vi "PyroAnalyze.vi"() -> ()   [LabVIEW 2014]
panel:
  out "Layer":i32
  out "Point":i32
  out "AllStacked":dbl[][][][](array[numeric])
  in  "Save Folder":path
  in  "StackAll":bool
  in  "Add":bool
  in  "Points":cluster{"X":dbl, "Y":dbl}[](array[cluster])
  in  "Size":u8
  in  "Save":bool
  in  "LayAvg":u16
  out "StackedAvg":u16[][][](array[numeric])
  in  "Stack":bool
  in  "Angle":dbl
  out "Image":dbl[][](graph)
  in  "ToImage":bool
  in  "NumPix":dbl
  in  "Width(mm)":dbl
  in  "Point1":cluster{"X":dbl, "Y":dbl}
  in  "Set1":bool
  out "Plot":cluster{"X":i16[], "Y":i16[]}(graph)
  in  "Deci":i32=5
  in  "Index":u32
  in  "Load":bool
  in  "Folder":path
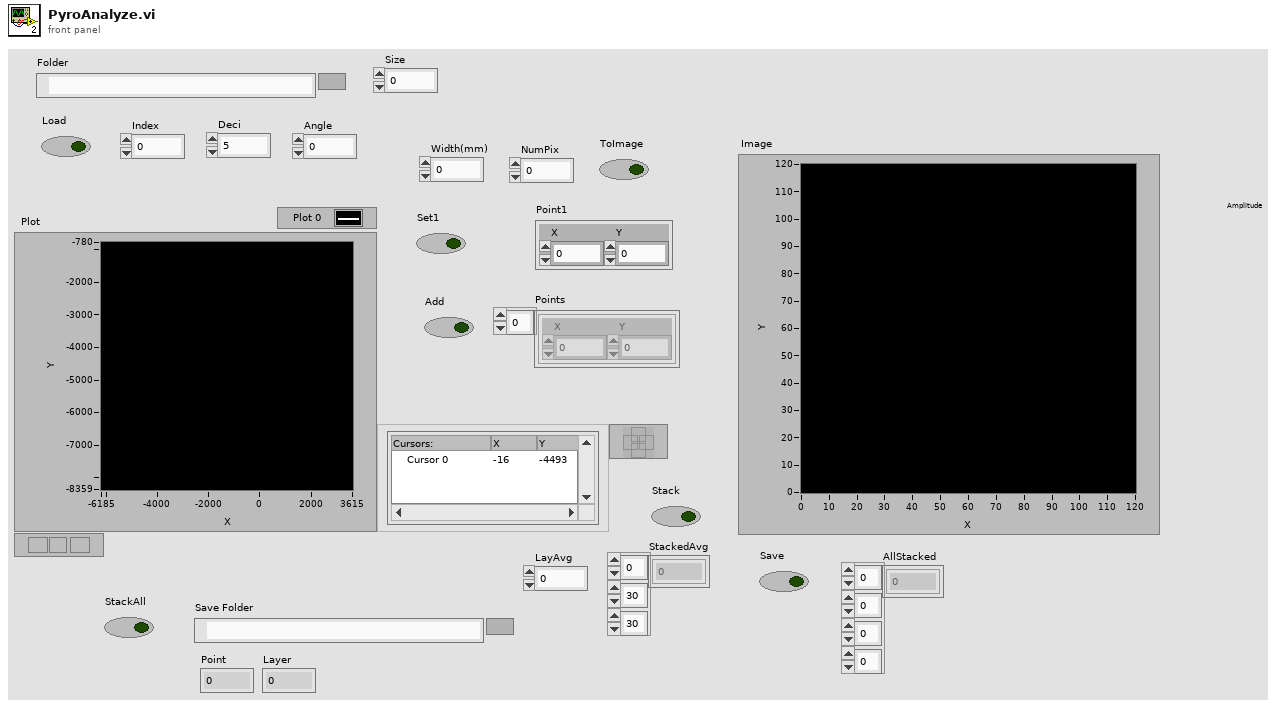
[diagram p1: front panel]
types:
  T1 = typedef "LVPointDoubleTypeDef.ctl" = cluster{"Cursor X":dbl, "Cursor Y":dbl}
  T2 = typedef "imagedata.ctl" = cluster{"image type":i32, "image depth":i32, "image":u8[], "mask":u8[], "colors":u32[], "Rectangle":cluster{"left":i16, "top":i16, "right":i16, "bottom":i16}}
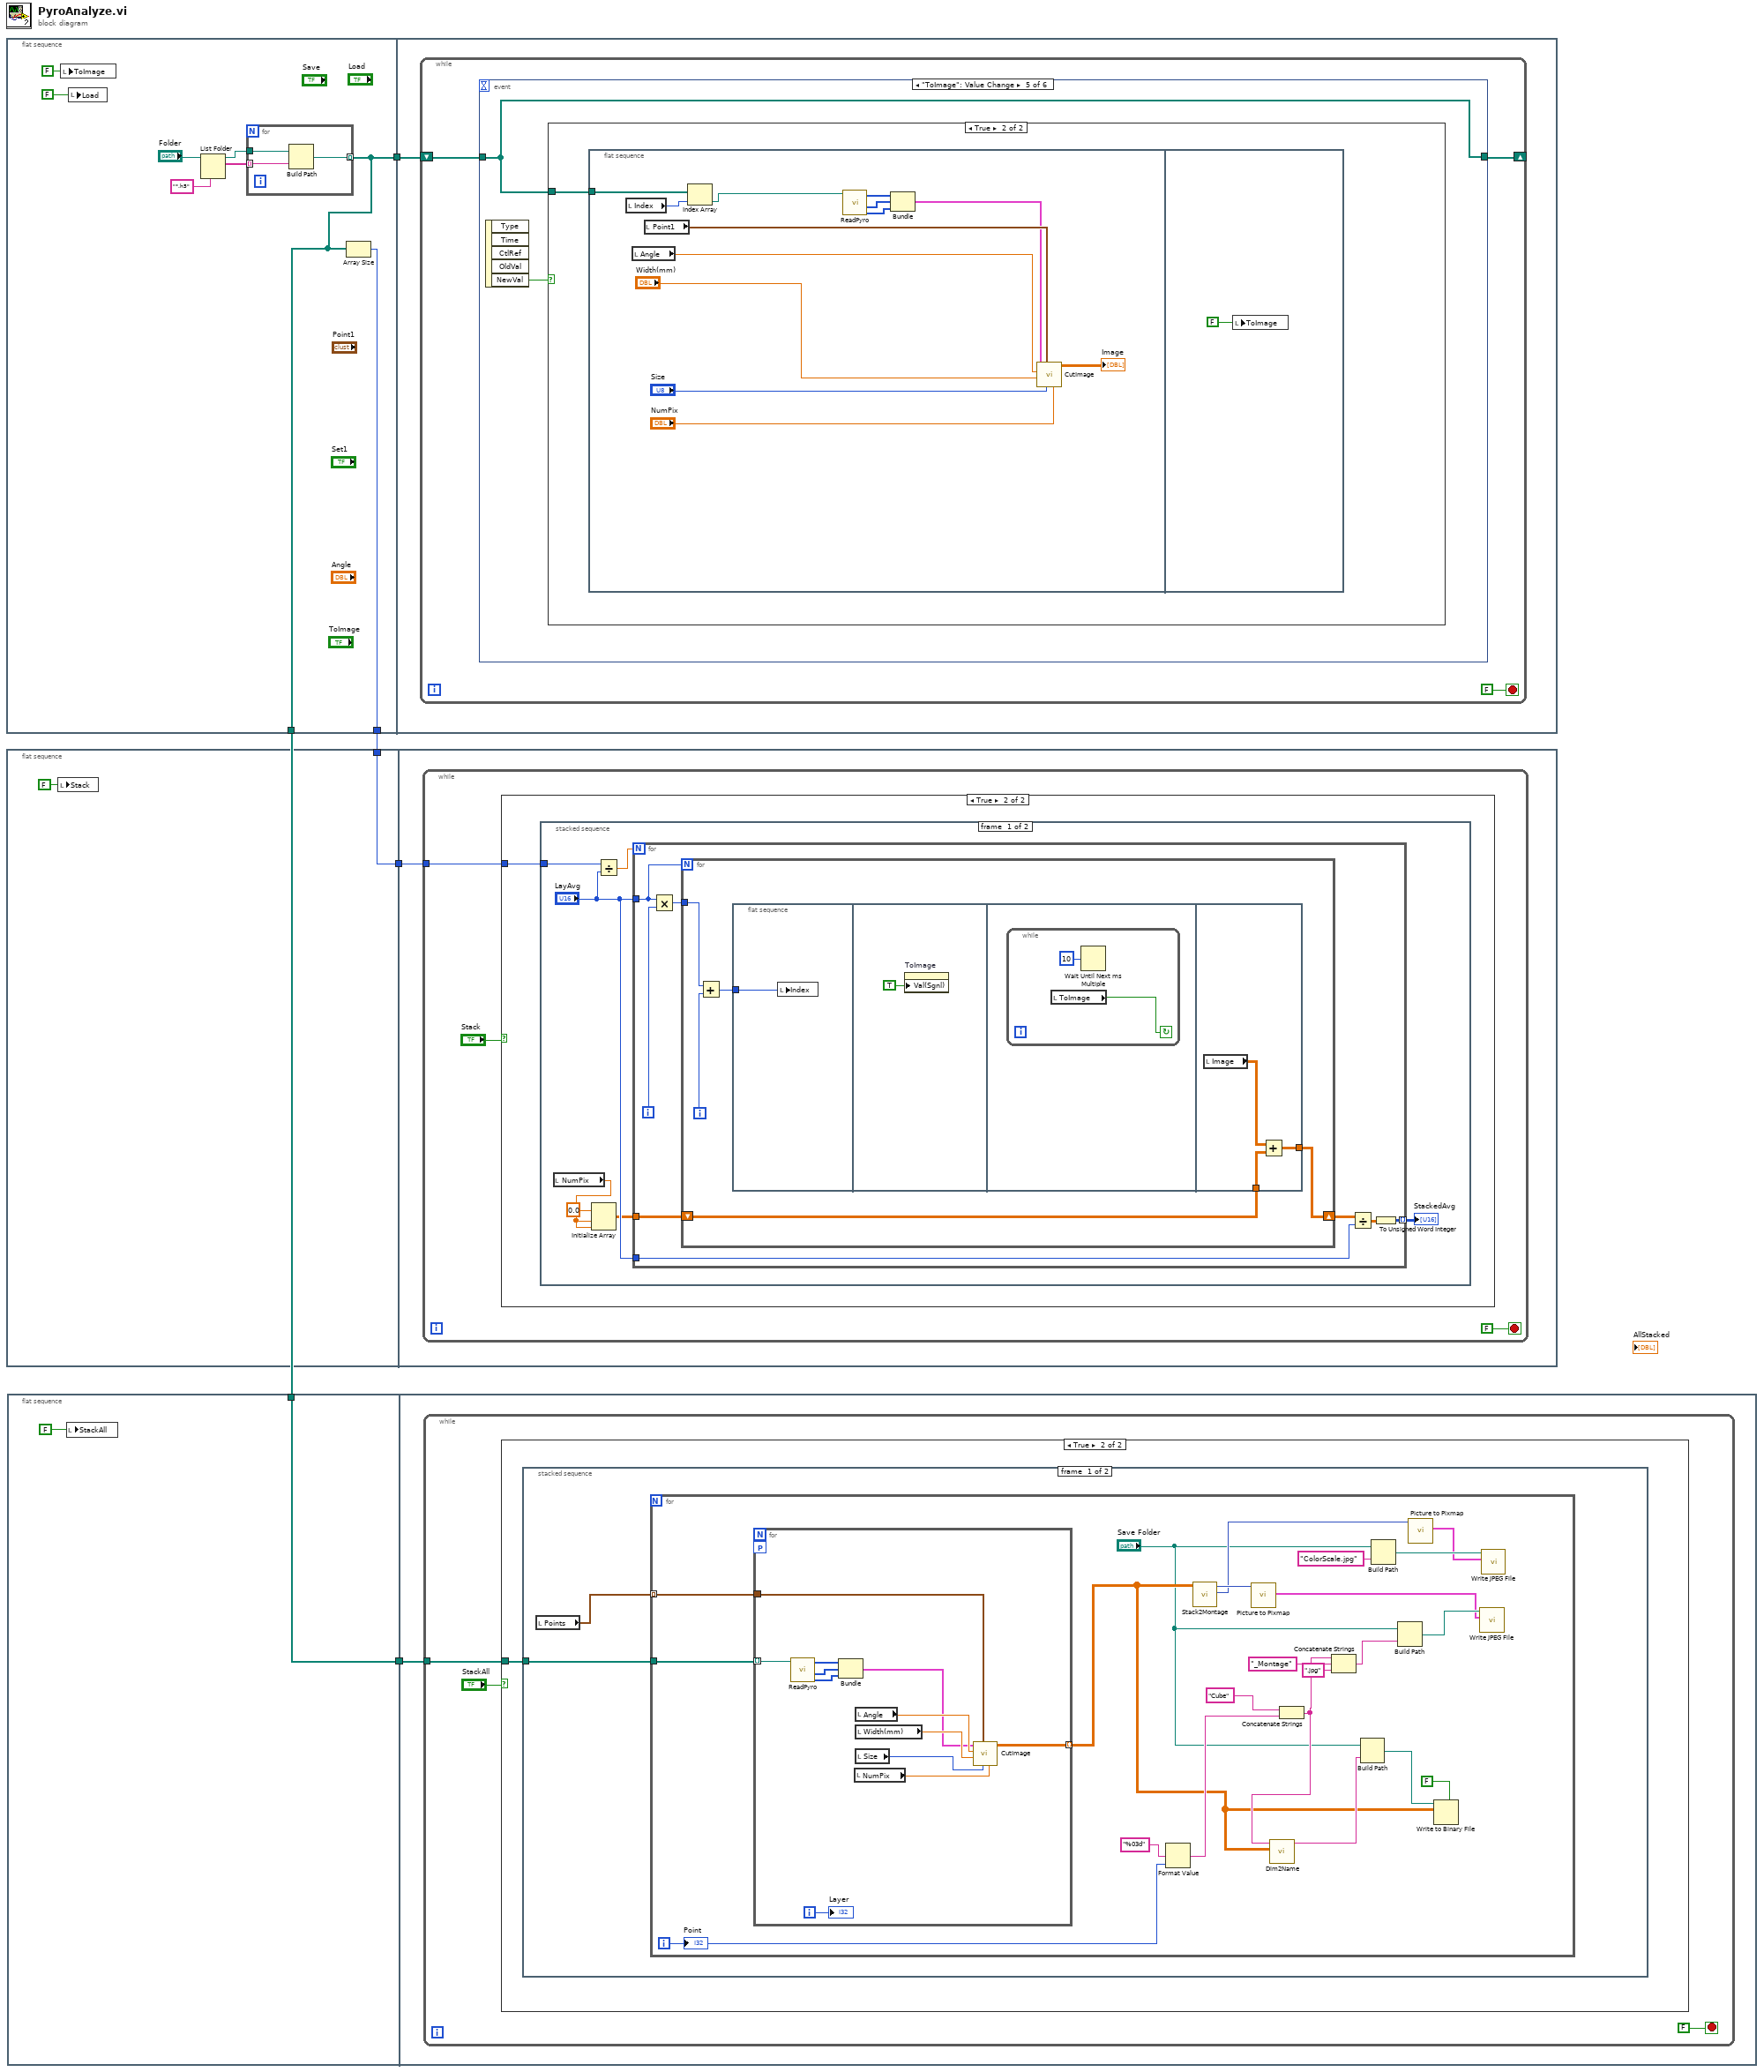
[diagram p0: block diagram]
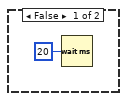
[diagram p2: hidden frame]
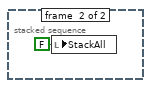
[diagram p3: hidden frame]
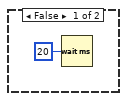
[diagram p4: hidden frame]
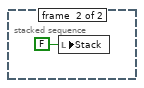
[diagram p5: hidden frame]
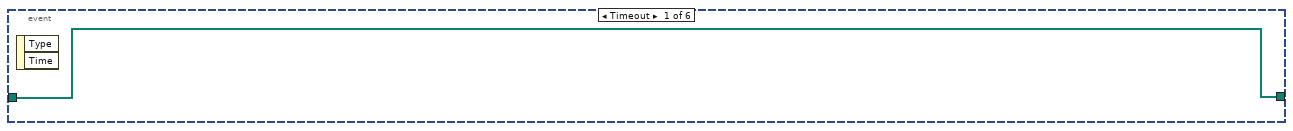
[diagram p6: hidden frame]
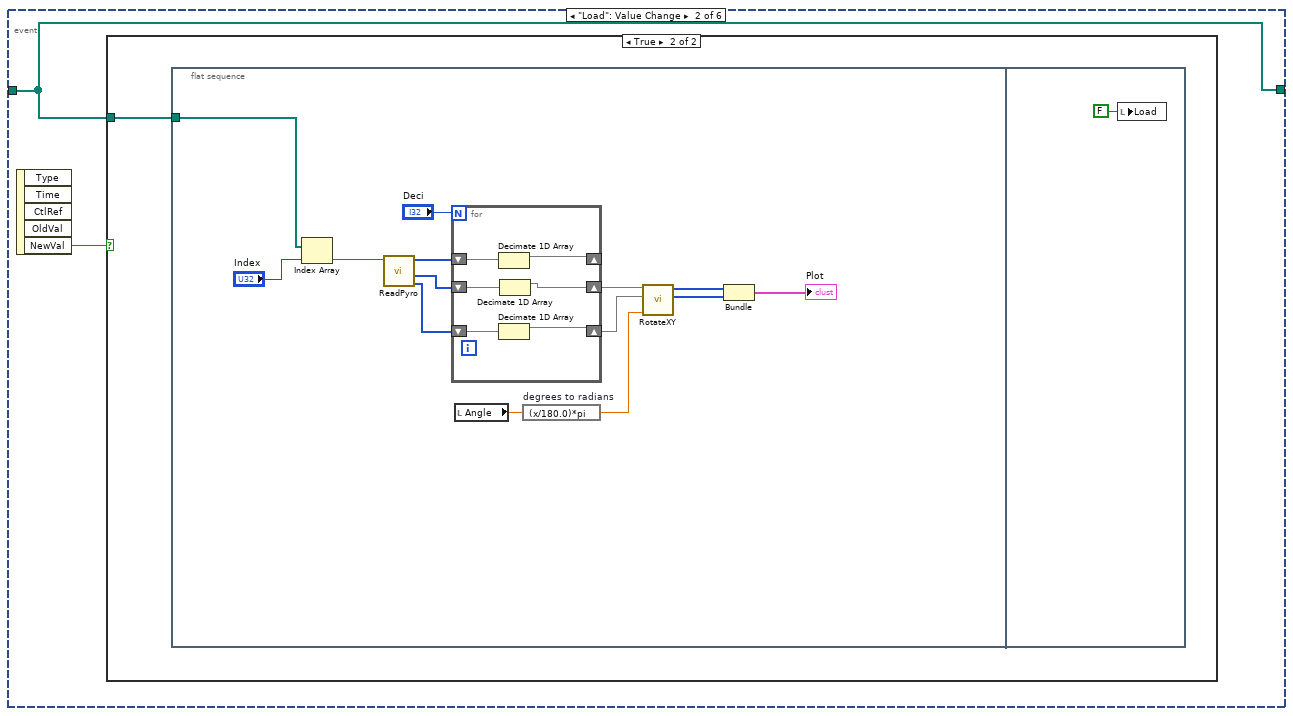
[diagram p7: hidden frame]
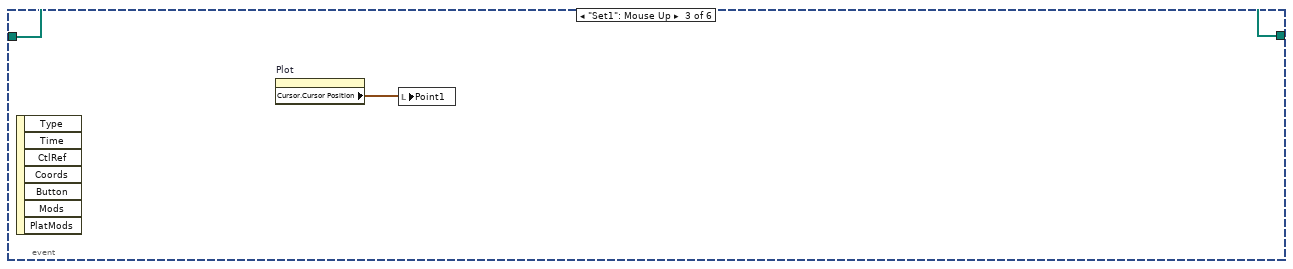
[diagram p9: hidden frame]
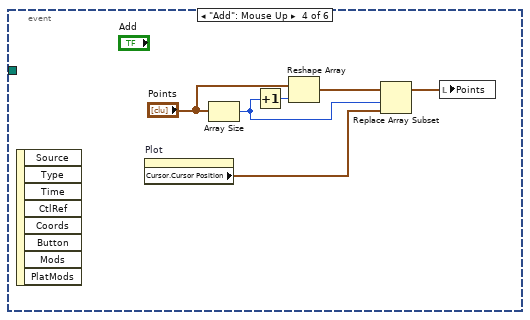
[diagram p10: hidden frame]
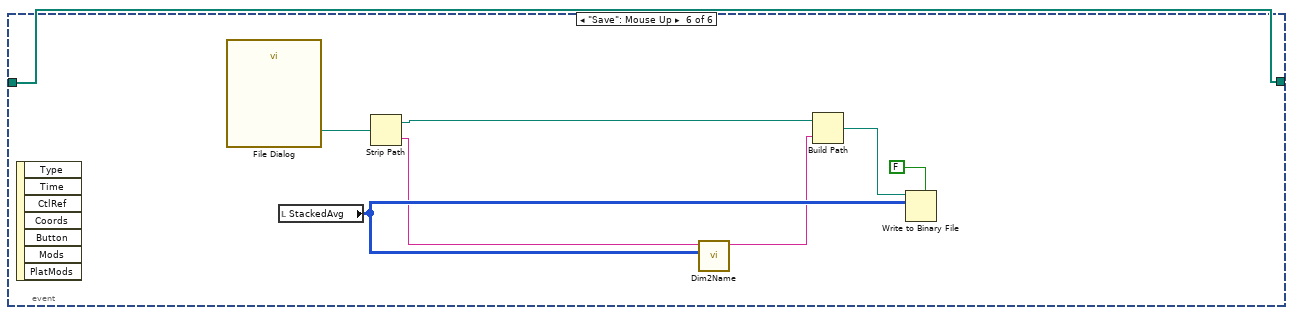
[diagram p12: hidden frame]
diagram:
  n1 = flat-sequence {
    tunnel: [w6] -> w5
    tunnel: [w7] -> w4
    tunnel: [w6] -> w2
    tunnel: w5 -> [w17]
    frame #0 {
      n2 = local write "ToImage"(FALSE ("ToImage")) -> ()
      n3 = local write "Load"(FALSE ("ToImage")) -> ()
      n4 = List Folder(path="Folder", pattern="*.h5") -> (path out=w10:path, filenames=w11:string[])  [unwired: 2 in, 2 out]
      n5 = for {
        tunnel: w11 -> [w16] mode=indexing
        tunnel: w10 -> [w15]
        tunnel: [w14] -> w6 mode=indexing
        n6 = Build Path(base path=w15, name or relative path=w16) -> (appended path=w14:path)
      }
      n7 = Array Size(array=w6) -> (size(s)=w7:i32)
    }
    frame #1 {
      n8 = while {
        shift-right: [w18] -> _
        shift-left: w17 -> [w19]
        stop <- FALSE stop-if-true
        n9 = event shown="[4] \"ToImage\": Value Change" {
          selector: _ -> [_ _ _ _ _ _]
          dyn-events: _ -> [_ _ _ _ _ _]
          timeout: _ -> [_ _ _ _ _ _]
          tunnel: w19 -> [w21 w23 w47 _ w54 w78]
          tunnel: [w21 w23 w47 _ w54 w78] -> w18
          event Timeout {
            n10 = event-data() -> ()  [unwired: 1 in, 2 out]
          }
          event "Load": Value Change {
            n11 = event-data() -> ("NewVal"=w22:bool)  [unwired: 1 in, 4 out]
            n12 = case shown="True" w22 {
              tunnel: w23 -> [_ w24]
              frame False {
              }
              frame True {
                n13 = flat-sequence {
                  tunnel: w24 -> [w32]
                  frame #0 {
                    n14 = Index Array(array=w32, index="Index") -> (element=w31:path)
                    n15 = call "ReadPyro.vi"("Path"=w31) -> ("Y"=w34:i16[], "X"=w35:i16[], "Pyro1"=w37:i16[])  [unwired: 6 in, 2 out]
                    n16 = for {
                      N: "Deci" -> [_]
                      shift-right: [w41] -> _
                      shift-left: w37 -> [w44]
                      shift-right: [w40] -> w30
                      shift-left: w35 -> [w43]
                      shift-right: [w39] -> w29
                      shift-left: w34 -> [w42]
                      n17 = Decimate 1D Array(w44) -> (w41:i16[])  [unwired: 1 out]
                      n18 = Decimate 1D Array(w42) -> (w39:i16[])  [unwired: 1 out]
                      n19 = Decimate 1D Array(w43) -> (w40:i16[])  [unwired: 1 out]
                    }
                    n20 = local read "Angle"() -> (w26:dbl)
                    n21 = expression code="(x/180.0)*pi" "degrees to radians"(w26) -> (w25:dbl)
                    n22 = call "RotateXY.vi"("Angle"=w25, "Y"=w29, "X"=w30) -> ("Yout"=w27:i16[], "Xout"=w28:i16[])  [unwired: 7 in]
                    n23 = Bundle("Xout"=w28, "Yout"=w27) -> (→"Plot":cluster{"Xout":i16[], "Yout":i16[]})  [unwired: 1 in]
                  }
                  frame #1 {
                    n24 = local write "Load"(FALSE ("Load")) -> ()
                  }
                }
              }
            }
          }
          event "Set1": Mouse Up {
            n25 = event-data() -> ()  [unwired: 1 in, 7 out]
            n26 = property on="Plot" class="XYGraph (strict)"() -> ("Cursor.Cursor Position"=w46:T1)  [unwired: 2 in, 2 out]
            n27 = local write "Point1"(w46) -> ()
          }
          event "Add": Mouse Up {
            n28 = event-data() -> ()  [unwired: 1 in, 8 out]
            n29 = property on="Plot" class="XYGraph (strict)"() -> ("Cursor.Cursor Position"=w53:T1)  [unwired: 2 in, 2 out]
            n30 = Array Size(array="Points") -> (size(s)=w48:i32)
            n31 = Increment(x=w48) -> (x+1=w49:i32)
            n32 = Reshape Array("Points", w49) -> (w50:cluster{"X":dbl, "Y":dbl}[])
            n33 = Replace Array Subset(array=w50, new element=w53, index=w48) -> (w52:cluster{"X":dbl, "Y":dbl}[])
            n34 = local write "Points"(w52) -> ()
          }
          event "ToImage": Value Change {
            n35 = event-data() -> ("NewVal"=w55:bool)  [unwired: 1 in, 4 out]
            n36 = case shown="True" w55 {
              tunnel: w54 -> [_ w56]
              frame False {
              }
              frame True {
                n37 = flat-sequence {
                  tunnel: w56 -> [w66]
                  frame #0 {
                    n38 = local read "Index"() -> (w65:u32)
                    n39 = local read "Angle"() -> (w69:dbl)
                    n40 = local read "Point1"() -> (w62:cluster{"X":dbl, "Y":dbl})
                    n41 = Index Array(array=w66, index=w65) -> (element=w58:path)
                    n42 = call "ReadPyro.vi"("Path"=w58) -> ("Y"=w59:i16[], "X"=w60:i16[], "Pyro1"=w61:i16[])  [unwired: 6 in, 2 out]
                    n43 = Bundle("Pyro1"=w61, "X"=w60, "Y"=w59) -> (w57:cluster{"Pyro1":i16[], "X":i16[], "Y":i16[]})  [unwired: 1 in]
                    n44 = call "CutImage.vi"("NumPix"="NumPix", "Size"="Size", "PointIn"=w62, "Width(mm)"="Width(mm)", "Angle"=w69, "PyroIn"=w57) -> ("Image"=→"Image":dbl[][])  [unwired: 5 in]
                  }
                  frame #1 {
                    n45 = local write "ToImage"(FALSE ("ToImage")) -> ()
                  }
                }
              }
            }
          }
          event "Save": Mouse Up {
            n46 = event-data() -> ()  [unwired: 1 in, 7 out]
            n47 = call "File Dialog"() -> ("selected path"=w76:path)  [unwired: 12 in, 3 out]
            n48 = local read "StackedAvg"() -> (w77:u16[][][])
            n49 = Strip Path(path=w76) -> (stripped path=w74:path, name=w75:string)
            n50 = call "Dim2Name.vi"("StackedAvg"=w77, "name"=w75) -> ("String"=w73:string)  [unwired: 9 in]
            n51 = Build Path(base path=w74, name or relative path=w73) -> (appended path=w72:path)
            n52 = Write to Binary File(file (use dialog)=w72, data=w77, 5:FALSE ("prepend array or string size? (T)")) -> ()  [unwired: 3 in, 3 out]
          }
        }
      }
    }
  }
  n53 = flat-sequence {
    tunnel: w4 -> [w79]
    tunnel: [w79] -> w3
    tunnel: w3 -> [w81]
    frame #0 {
      n54 = local write "Stack"(FALSE ("Stack")) -> ()
    }
    frame #1 {
      n55 = while {
        tunnel: w81 -> [w82]
        stop <- FALSE stop-if-true
        n56 = case shown="True" "Stack" {
          tunnel: w82 -> [_ w86]
          frame False {
            n57 = Wait (ms)(milliseconds to wait=u32 20) -> ()  [unwired: 1 out]
          }
          frame True {
            n58 = stacked-sequence {
              tunnel: w86 -> [w93 _]
              frame #0 {
                n59 = local read "NumPix"() -> (w89:dbl)
                n60 = Initialize Array(0.0 ("element"), w89, w89) -> (w87:dbl[][])
                n61 = Divide(x=w93, y="LayAvg") -> (x/y=w92:dbl)
                n62 = for {
                  N: w92 -> [_]
                  tunnel: "LayAvg" -> [w94]
                  tunnel: w87 -> [w99]
                  tunnel: "LayAvg" -> [w97]
                  tunnel: [w95] -> w90 mode=indexing
                  i -> [w101]
                  n63 = Multiply(x=w94, y=w101) -> (x*y=w100:i32)
                  n64 = for {
                    N: w94 -> [_]
                    tunnel: w100 -> [w106]
                    shift-right: [w102] -> w98
                    shift-left: w99 -> [w103]
                    i -> [w105]
                    n65 = Add(x=w106, y=w105) -> (x+y=w104:i32)
                    n66 = flat-sequence {
                      tunnel: w104 -> [w107]
                      tunnel: w103 -> [w113]
                      tunnel: [w111] -> w102
                      frame #0 {
                        n67 = local write "Index"(w107) -> ()
                      }
                      frame #1 {
                        n68 = property on="ToImage" class="Bool (strict)"("Val(Sgnl)"=TRUE ("Load")) -> ()  [unwired: 2 in, 2 out]
                      }
                      frame #2 {
                        n69 = while {
                          stop <- w110 continue-if-true
                          n70 = local read "ToImage"() -> (w110:bool)
                          n71 = Wait Until Next ms Multiple(millisecond multiple=u32 10) -> ()  [unwired: 1 out]
                        }
                      }
                      frame #3 {
                        n72 = local read "Image"() -> (w112:dbl[][])
                        n73 = Add(x=w112, y=w113) -> (x+y=w111:dbl[][])
                      }
                    }
                  }
                  n74 = Divide(x=w98, y=w97) -> (x/y=w96:dbl[][])
                  n75 = To Unsigned Word Integer(number=w96) -> (unsigned 16bit integer=w95:u16[][])
                }
                "StackedAvg" <- w90
              }
              frame #1 {
                n76 = local write "Stack"(FALSE ("Stack")) -> ()
              }
            }
          }
        }
      }
    }
  }
  n77 = flat-sequence {
    tunnel: w2 -> [w115]
    tunnel: [w115] -> w1
    tunnel: w1 -> [w117]
    frame #0 {
      n78 = local write "StackAll"(FALSE ("Stack")) -> ()
    }
    frame #1 {
      n79 = while {
        tunnel: w117 -> [w118]
        stop <- FALSE stop-if-true
        n80 = case shown="True" "StackAll" {
          tunnel: w118 -> [_ w122]
          frame False {
            n81 = Wait (ms)(milliseconds to wait=u32 20) -> ()  [unwired: 1 out]
          }
          frame True {
            n82 = stacked-sequence {
              tunnel: w122 -> [w123 _]
              frame #0 {
                n83 = local read "Points"() -> (w124:cluster{"X":dbl, "Y":dbl}[])
                n84 = for {
                  tunnel: w124 -> [w146] mode=indexing
                  tunnel: w123 -> [w145]
                  i -> [w130]
                  n85 = for {
                    tunnel: w146 -> [w158]
                    tunnel: [w153] -> w131 mode=indexing
                    tunnel: w145 -> [w148] mode=indexing
                    workers-P: _ -> [_]
                    i -> [w152]
                    n86 = call "ReadPyro.vi"("Path"=w148) -> ("Y"=w151:i16[], "X"=w150:i16[], "Pyro1"=w149:i16[])  [unwired: 6 in, 2 out]
                    n87 = Bundle("Pyro1"=w149, "X"=w150, "Y"=w151) -> (w147:cluster{"Pyro1":i16[], "X":i16[], "Y":i16[]})  [unwired: 1 in]
                    n88 = local read "NumPix"() -> (w154:dbl)
                    n89 = local read "Angle"() -> (w157:dbl)
                    n90 = local read "Width(mm)"() -> (w156:dbl)
                    n91 = local read "Size"() -> (w155:u8)
                    n92 = call "CutImage.vi"("NumPix"=w154, "Size"=w155, "PointIn"=w158, "Width(mm)"=w156, "Angle"=w157, "PyroIn"=w147) -> ("Image"=w153:dbl[][])  [unwired: 5 in]
                    "Layer" <- w152
                  }
                  n93 = Format Value(format string="%03d", value (0)=w130) -> (output string=w143:string)  [unwired: 1 in]
                  n94 = call "Stack2Montage.vi"("StackedAvg"=w131) -> ("ColorScale"=w126:picture, "Montage"=w134:picture)  [unwired: 9 in]
                  n95 = call <vilib>:"Picture to Pixmap.vi"("picture"=w134) -> ("image data"=w133:T2)  [unwired: 9 in, 1 out]
                  n96 = Concatenate Strings("Cube" ("string"), w143) -> (w138:string)
                  n97 = call "Dim2Name.vi"("StackedAvg"=w131, "name"=w138) -> ("String"=w140:string)  [unwired: 9 in]
                  n98 = Concatenate Strings(w138, "_Montage" ("string"), ".jpg" ("string")) -> (w136:string)
                  n99 = Build Path(base path="Save Folder", name or relative path=w140) -> (appended path=w141:path)
                  n100 = Build Path(base path="Save Folder", name or relative path="ColorScale.jpg") -> (appended path=w128:path)
                  n101 = Build Path(base path="Save Folder", name or relative path=w136) -> (appended path=w135:path)
                  n102 = call <vilib>:"Picture to Pixmap.vi"("picture"=w126) -> ("image data"=w127:T2)  [unwired: 9 in, 1 out]
                  n103 = Write to Binary File(file (use dialog)=w141, data=w131, 5:FALSE ("prepend array or string size? (T)")) -> ()  [unwired: 3 in, 3 out]
                  n104 = call <vilib>:"Write JPEG File.vi"("image data"=w133, "path to JPEG file"=w135) -> ()  [unwired: 8 in, 2 out]
                  n105 = call <vilib>:"Write JPEG File.vi"("image data"=w127, "path to JPEG file"=w128) -> ()  [unwired: 8 in, 2 out]
                  "Point" <- w130
                }
              }
              frame #1 {
                n106 = local write "StackAll"(FALSE ("Stack")) -> ()
              }
            }
          }
        }
      }
    }
  }
